vi "Terminal-Main-DeviceLubricateUnit.vi"(4 "ErrorQRef":refnum<queue>, 5 "ModbusNResRef":refnum<notifier>, 6 "ModbusMsgQRef":refnum<queue>, 7 "ModbusNReqRef":refnum<notifier>, 8 "error in (no error)":errorcluster caption="错误输入（无错误）", 11 "DeviceLubricateUnitNRef":refnum<notifier>) -> (0 "error out":errorcluster caption="错误输出")   [LabVIEW 2014]
panel:
  out "Device Lubricate Unit is running":bool
  out "DeviceLubricateUnit开始通知器":refnum<notifier>
  out "DeviceLubricateUnit开始响应器":refnum<notifier>
  out "DeviceLubricateUnit停止通知器":refnum<notifier>
  out "DeviceLubricateUnit停止响应器":refnum<notifier>
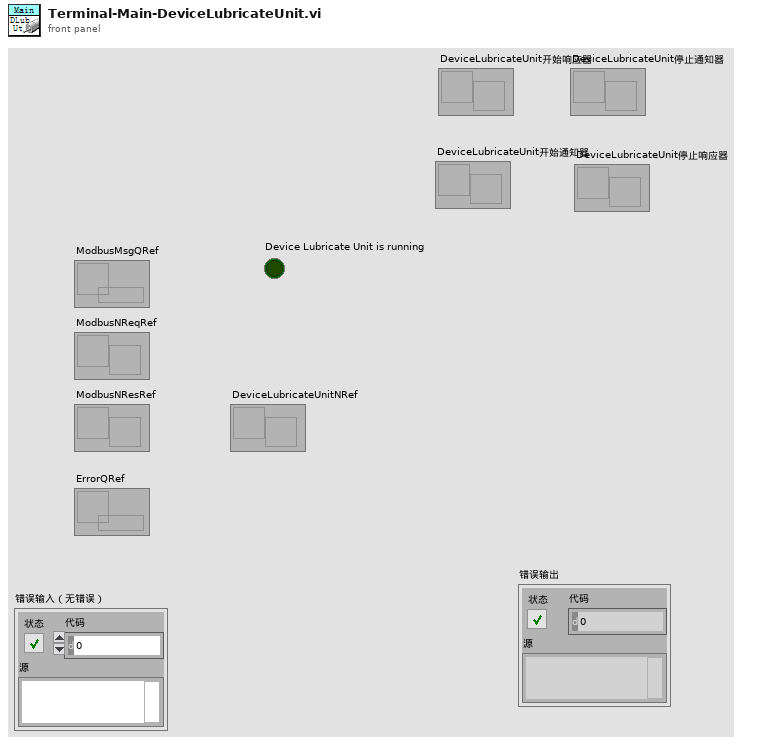
[diagram p1: front panel]
types:
  T1 = cluster{"Transaction ID":u16, "Unit ID":u8, "Starting Address":u16, "Quantity":u16}
  T2 = cluster{"Transaction ID":u16, "Unit ID":u8, "Address":u16, "Register":u16}
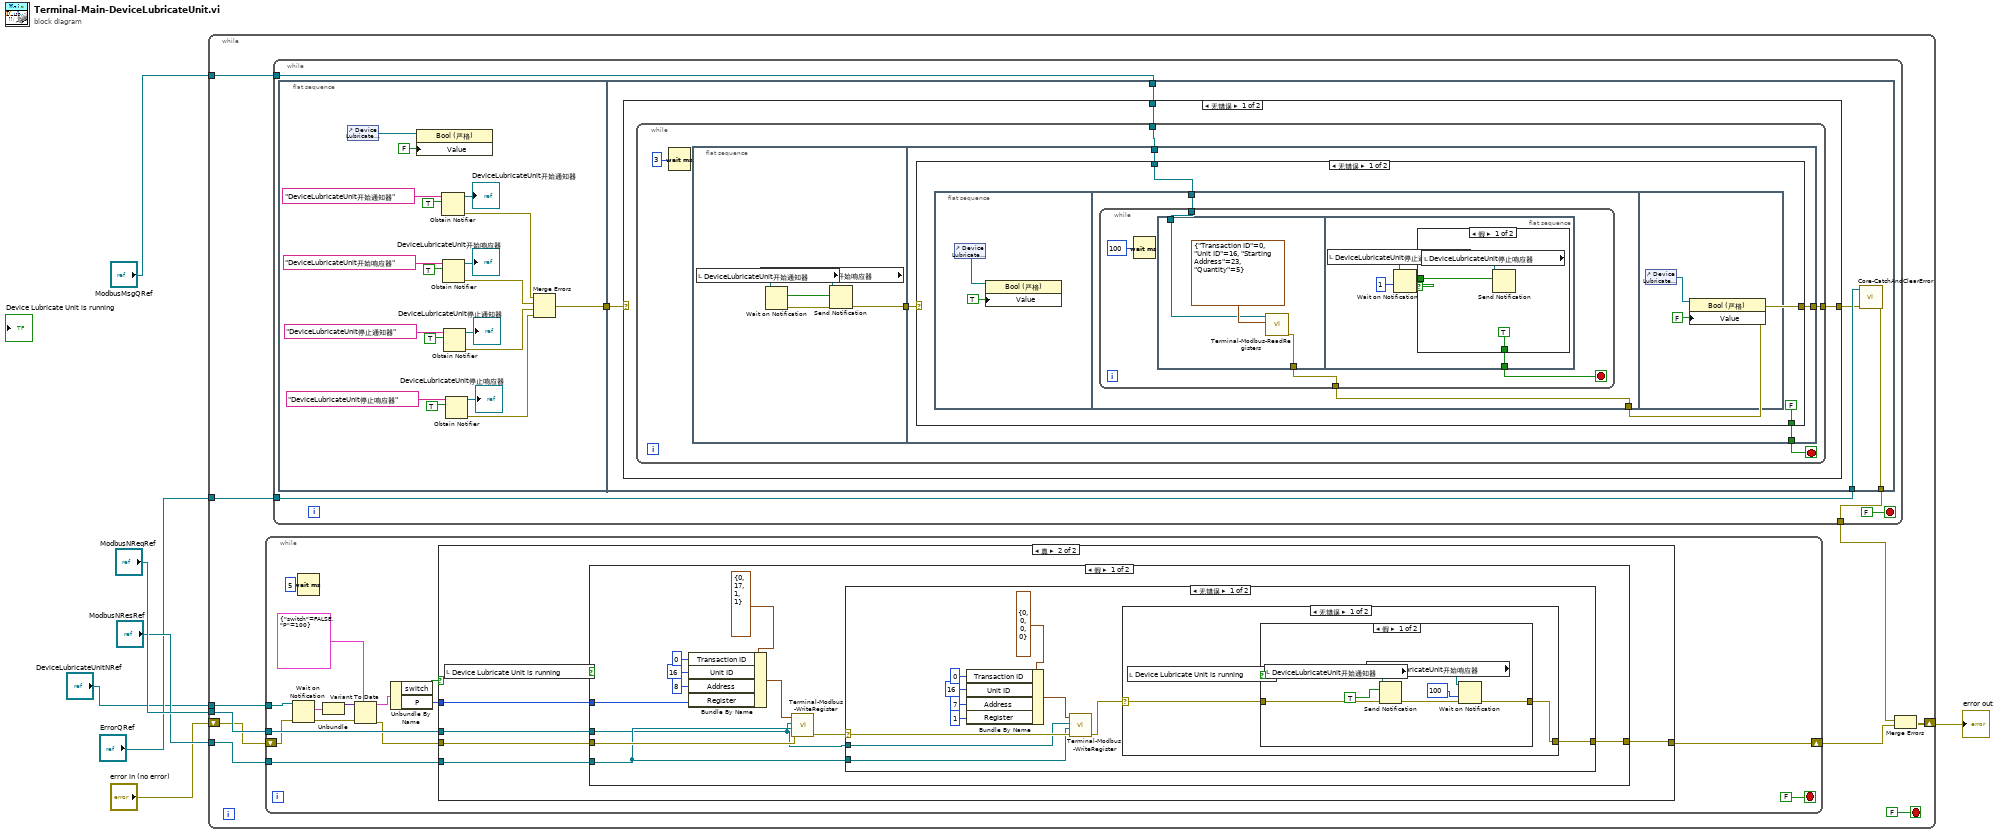
[diagram p0: block diagram]
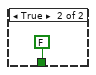
[diagram p2: hidden frame]
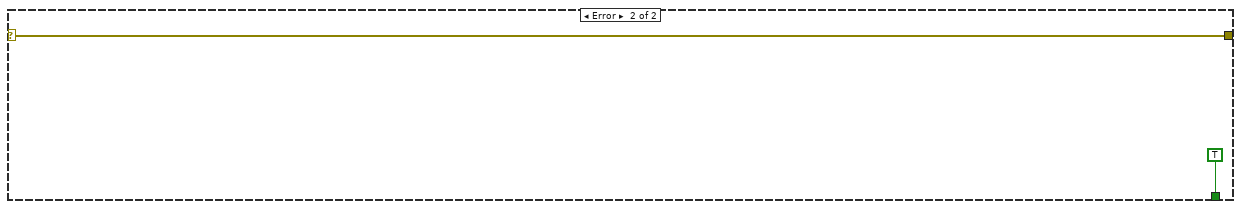
[diagram p3: hidden frame]
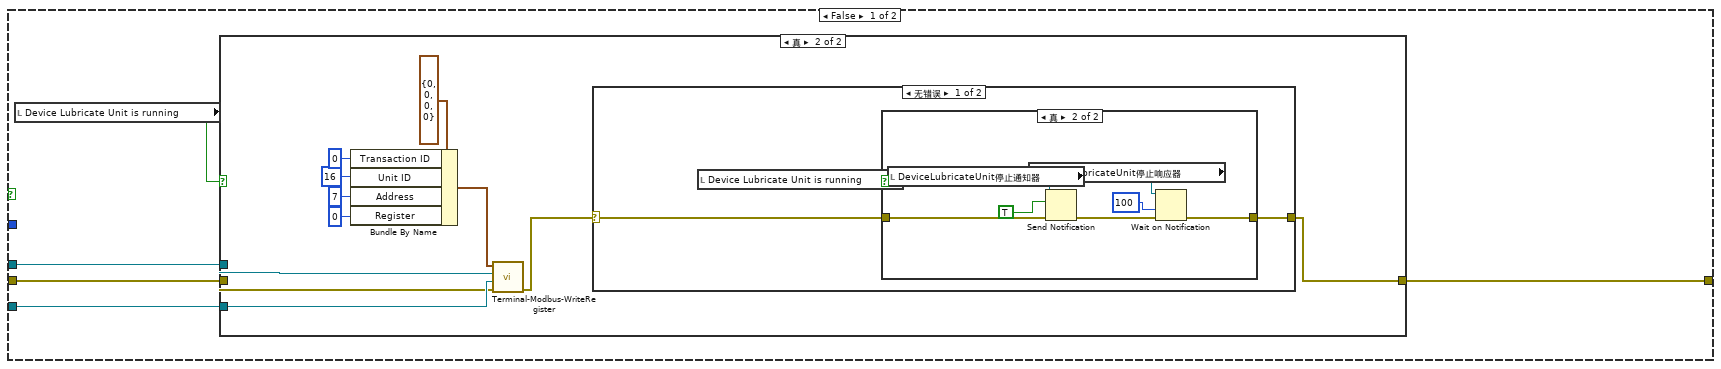
[diagram p5: hidden frame]
diagram:
  n1 = while {
    tunnel: "ModbusMsgQRef" -> [w17]
    tunnel: "ModbusNReqRef" -> [w16]
    tunnel: "ModbusNResRef" -> [w15]
    tunnel: "ErrorQRef" -> [w13]
    shift-right: [w12] -> w2
    shift-left: "error in (no error)" -> [w14]
    tunnel: "DeviceLubricateUnitNRef" -> [w8]
    stop <- FALSE stop-if-true
    n2 = while {
      tunnel: w16 -> [w105]
      tunnel: w15 -> [w104]
      shift-right: [w103] -> w11
      shift-left: w14 -> [w99]
      tunnel: w8 -> [w100]
      stop <- FALSE stop-if-true
      n3 = Wait on Notification(notifier=w100, error in (no error)=w99) -> (notification=w98:cluster{variant, string}, error out=w94:errorcluster)  [unwired: 2 in, 2 out]
      n4 = Wait (ms)(milliseconds to wait=u32 5 ("等待时间（毫秒）")) -> ()  [unwired: 1 out]
      n5 = Unbundle(w98) -> (w97:variant)  [unwired: 1 out]
      n6 = Variant To Data(error in=w94, type=cluster{"switch":bool, "P":u16} {"switch"=FALSE, "P"=100}, Variant=w97) -> (data=w96:cluster{"switch":bool, "P":u16}, error out=w93:errorcluster)
      n7 = Unbundle By Name(w96) -> ("switch"=w95:bool, "P"=w91:u16)
      n8 = case shown="真" w95 {
        tunnel: w105 -> [w110 w138]
        tunnel: w104 -> [w109 w139]
        tunnel: w93 -> [w108 w140]
        tunnel: [w107 w137] -> w103
        tunnel: w91 -> [_ w135]
        frame False {
          n9 = local read "Device Lubricate Unit is running"() -> (w106:bool)
          n10 = case shown="真" w106 {
            tunnel: w110 -> [_ w121]
            tunnel: w109 -> [_ w120]
            tunnel: w108 -> [w111 w119]
            tunnel: [w111 w118] -> w107
            frame False {
            }
            frame True {
              n11 = Bundle By Name(cluster=T2 {"Transaction ID"=0, "Unit ID"=0, "Address"=0, "Register"=0} ("簇"), "Transaction ID"=u16 0, "Unit ID"=u8 16, "Address"=u16 7, "Register"=u16 0) -> (w113:T2)
              n12 = call "Terminal-Modbus-WriteRegister.vi"("error in (no error)"=w119, "ModbusNResRef"=w120, "ModbusNReqRef"=w121, "簇"=w113) -> ("error out"=w122:errorcluster)  [unwired: 7 in]
              n13 = case shown="无错误" w122 {
                selector: w122 -> [w124 w134]
                tunnel: [w123 w134] -> w118
                frame No Error {
                  n14 = local read "Device Lubricate Unit is running"() -> (w125:bool)
                  n15 = case shown="真" w125 {
                    tunnel: [w126 w128] -> w123
                    tunnel: w124 -> [w126 w127]
                    frame False {
                    }
                    frame True {
                      n16 = local read "DeviceLubricateUnit停止通知器"() -> (w133:refnum<notifier>)
                      n17 = local read "DeviceLubricateUnit停止响应器"() -> (w130:refnum<notifier>)
                      n18 = Send Notification(notification=TRUE ("通知"), notifier=w133, error in (no error)=w127) -> (error out=w131:errorcluster)  [unwired: 1 out]
                      n19 = Wait on Notification(notifier=w130, timeout in ms (-1)=100 ("超时毫秒(-1)"), error in (no error)=w131) -> (error out=w128:errorcluster)  [unwired: 1 in, 3 out]
                    }
                  }
                }
                frame Error {
                }
              }
            }
          }
        }
        frame True {
          n20 = local read "Device Lubricate Unit is running"() -> (w136:bool)
          n21 = case shown="假" w136 {
            tunnel: w140 -> [w150 w176]
            tunnel: w139 -> [w142 _]
            tunnel: w138 -> [w141 _]
            tunnel: [w149 w176] -> w137
            tunnel: w135 -> [w148 _]
            frame False {
              n22 = Bundle By Name(cluster=T2 {"Transaction ID"=0, "Unit ID"=17, "Address"=1, "Register"=1} ("簇"), "Transaction ID"=u16 0, "Unit ID"=u8 16, "Address"=u16 8, "Register"=w148) -> (w144:T2)
              n23 = call "Terminal-Modbus-WriteRegister.vi"("error in (no error)"=w150, "ModbusNResRef"=w142, "ModbusNReqRef"=w141, "簇"=w144) -> ("error out"=w151:errorcluster)  [unwired: 7 in]
              n24 = case shown="无错误" w151 {
                selector: w151 -> [w161 w175]
                tunnel: w141 -> [w160 _]
                tunnel: w142 -> [w159 _]
                tunnel: [w158 w175] -> w149
                frame No Error {
                  n25 = Bundle By Name(cluster=T2 {"Transaction ID"=0, "Unit ID"=0, "Address"=0, "Register"=0} ("簇"), "Transaction ID"=u16 0, "Unit ID"=u8 16, "Address"=u16 7, "Register"=u16 1) -> (w153:T2)
                  n26 = call "Terminal-Modbus-WriteRegister.vi"("error in (no error)"=w161, "ModbusNResRef"=w159, "ModbusNReqRef"=w160, "簇"=w153) -> ("error out"=w162:errorcluster)  [unwired: 7 in]
                  n27 = case shown="无错误" w162 {
                    selector: w162 -> [w164 w174]
                    tunnel: [w163 w174] -> w158
                    frame No Error {
                      n28 = local read "Device Lubricate Unit is running"() -> (w165:bool)
                      n29 = case shown="假" w165 {
                        tunnel: [w167 w173] -> w163
                        tunnel: w164 -> [w166 w173]
                        frame False {
                          n30 = local read "DeviceLubricateUnit开始通知器"() -> (w172:refnum<notifier>)
                          n31 = local read "DeviceLubricateUnit开始响应器"() -> (w169:refnum<notifier>)
                          n32 = Send Notification(notification=TRUE ("通知"), notifier=w172, error in (no error)=w166) -> (error out=w170:errorcluster)  [unwired: 1 out]
                          n33 = Wait on Notification(notifier=w169, timeout in ms (-1)=100 ("超时毫秒(-1)"), error in (no error)=w170) -> (error out=w167:errorcluster)  [unwired: 1 in, 3 out]
                        }
                        frame True {
                        }
                      }
                    }
                    frame Error {
                    }
                  }
                }
                frame Error {
                }
              }
            }
            frame True {
            }
          }
        }
      }
    }
    n34 = while {
      tunnel: w17 -> [w21]
      tunnel: w13 -> [w20]
      tunnel: [w18] -> w10
      stop <- FALSE stop-if-true
      n35 = flat-sequence {
        tunnel: [w24] -> w22
        tunnel: w22 -> [w46]
        tunnel: w20 -> [w45]
        tunnel: [w43] -> w18
        tunnel: w21 -> [w42]
        frame #0 {
          n36 = control-ref of="Device Lubricate Unit is running"() -> (w23:refnum<vi>)
          n37 = property class="Bool (严格)"(reference=w23, "Value"=FALSE ("值")) -> ()  [unwired: 1 in, 2 out]
          n38 = Obtain Notifier(name (unnamed)="DeviceLubricateUnit开始通知器" ("名称（未命名）"), notification data type=TRUE) -> (notifier out=→"DeviceLubricateUnit开始通知器":refnum<notifier>, error out=w28:errorcluster)  [unwired: 2 in, 1 out]
          n39 = Obtain Notifier(name (unnamed)="DeviceLubricateUnit开始响应器" ("名称（未命名）"), notification data type=TRUE) -> (notifier out=→"DeviceLubricateUnit开始响应器":refnum<notifier>, error out=w27:errorcluster)  [unwired: 2 in, 1 out]
          n40 = Obtain Notifier(name (unnamed)="DeviceLubricateUnit停止通知器" ("名称（未命名）"), notification data type=TRUE) -> (notifier out=→"DeviceLubricateUnit停止通知器":refnum<notifier>, error out=w26:errorcluster)  [unwired: 2 in, 1 out]
          n41 = Obtain Notifier(name (unnamed)="DeviceLubricateUnit停止响应器" ("名称（未命名）"), notification data type=TRUE) -> (notifier out=→"DeviceLubricateUnit停止响应器":refnum<notifier>, error out=w25:errorcluster)  [unwired: 2 in, 1 out]
          n42 = Merge Errors(w28, w27, w26, w25) -> (w24:errorcluster)
        }
        frame #1 {
          n43 = case shown="无错误" w46 {
            selector: w46 -> [_ w90]
            tunnel: [w48 w90] -> w44
            tunnel: w42 -> [w47 _]
            frame No Error {
              n44 = while {
                tunnel: [w51] -> w48
                tunnel: w47 -> [w50]
                stop <- w52 stop-if-true
                n45 = Wait (ms)(milliseconds to wait=u32 3 ("等待时间（毫秒）")) -> ()  [unwired: 1 out]
                n46 = flat-sequence {
                  tunnel: [w54] -> w53
                  tunnel: w53 -> [w62]
                  tunnel: [w61] -> w52
                  tunnel: [w60] -> w51
                  tunnel: w50 -> [w59]
                  frame #0 {
                    n47 = local read "DeviceLubricateUnit开始通知器"() -> (w58:refnum<notifier>)
                    n48 = local read "DeviceLubricateUnit开始响应器"() -> (w57:refnum<notifier>)
                    n49 = Wait on Notification(notifier=w58) -> (notification=w55:bool, error out=w56:errorcluster)  [unwired: 3 in, 2 out]
                    n50 = Send Notification(notification=w55, notifier=w57, error in (no error)=w56) -> (error out=w54:errorcluster)  [unwired: 1 out]
                  }
                  frame #1 {
                    n51 = case shown="无错误" w62 {
                      selector: w62 -> [_ w88]
                      tunnel: [FALSE TRUE] -> w61
                      tunnel: [w64 w88] -> w60
                      tunnel: w59 -> [w63 _]
                      frame No Error {
                        n52 = flat-sequence {
                          tunnel: [w68] -> w64
                          tunnel: w63 -> [w69]
                          frame #0 {
                            n53 = control-ref of="Device Lubricate Unit is running"() -> (w66:refnum<vi>)
                            n54 = property class="Bool (严格)"(reference=w66, "Value"=TRUE ("值")) -> ()  [unwired: 1 in, 2 out]
                          }
                          frame #1 {
                            n55 = while {
                              tunnel: w69 -> [w73]
                              tunnel: [w72] -> w68
                              stop <- w71 stop-if-true
                              n56 = Wait (ms)(milliseconds to wait=u32 100 ("等待时间（毫秒）")) -> ()  [unwired: 1 out]
                              n57 = flat-sequence {
                                tunnel: w73 -> [w75]
                                tunnel: [w74] -> w72
                                tunnel: [w77] -> w71
                                frame #0 {
                                n58 = call "Terminal-Modbus-ReadRegisters.vi"("簇"=T1 {"Transaction ID"=0, "Unit ID"=16, "Starting Address"=23, "Quantity"=5}, "ModbusMsgQRef"=w75) -> ("error out"=w74:errorcluster)  [unwired: 9 in]
                                }
                                frame #1 {
                                n59 = local read "DeviceLubricateUnit停止通知器"() -> (w80:refnum<notifier>)
                                n60 = Wait on Notification(notifier=w80, timeout in ms (-1)=1 ("超时毫秒(-1)")) -> (notification=w78:bool, timed out?=w79:bool)  [unwired: 2 in, 2 out]
                                n61 = case shown="假" w79 {
                                tunnel: [TRUE FALSE] -> w77
                                tunnel: w78 -> [w83 _]
                                frame False {
                                n62 = local read "DeviceLubricateUnit停止响应器"() -> (w82:refnum<notifier>)
                                n63 = Send Notification(notification=w83, notifier=w82) -> ()  [unwired: 1 in, 2 out]
                                }
                                frame True {
                                }
                                }
                                }
                              }
                            }
                          }
                          frame #2 {
                            n64 = control-ref of="Device Lubricate Unit is running"() -> (w86:refnum<vi>)
                            n65 = property class="Bool (严格)"(reference=w86, "Value"=FALSE ("值")) -> ()  [unwired: 1 in, 2 out]
                          }
                        }
                      }
                      frame Error {
                      }
                    }
                  }
                }
              }
            }
            frame Error {
            }
          }
          n66 = call "Core-CatchAndClearError.vi"("error in (no error)"=w44, "ErrorQ"=w45) -> ("error out"=w43:errorcluster)  [unwired: 7 in]
        }
      }
    }
    n67 = Merge Errors(w10, w11) -> (w12:errorcluster)
  }
  "error out" <- w2
